vi "Action.vi"(8 "error in (no error)":errorcluster, 10 "Actor in":refnum<class "Tamagotchi Basic Actor.lvclass">, 11 "Sleep Message in":refnum<class "Sleep Message.lvclass">) -> (0 "error out":errorcluster, 2 "Actor out":refnum<class "Tamagotchi Basic Actor.lvclass">, 3 "Sleep Message out":refnum<class "Sleep Message.lvclass">)   [LabVIEW 2026, in "Sleep Message.lvclass"]
uses:
  Sleep Message.lvclass
  Tamagotchi Basic Actor/Tamagotchi Basic Actor.lvclass
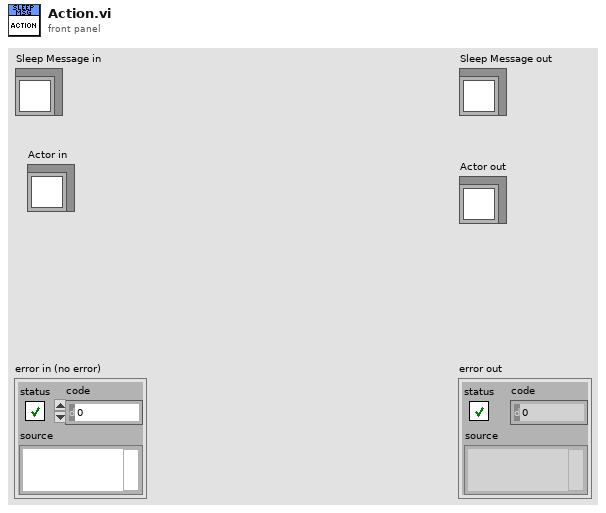
[diagram p1: front panel]
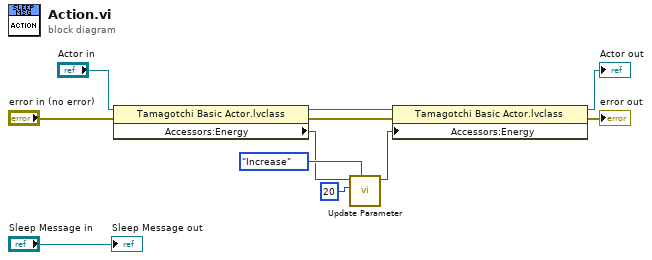
[diagram p0: block diagram]
diagram:
  n1 = property class="Tamagotchi Basic Actor.lvclass"(reference="Actor in", error in="error in (no error)") -> (reference out=w7:refnum<class "Tamagotchi Basic Actor.lvclass">, error out=w1:errorcluster, "Accessors:Energy"=w5:i16)
  n2 = call "Update Parameter.vi"("Action"=enum16{"Increase", "Decrease"}."Increase", "Modifier"=i16 20 ("y"), "Parameter"=w5) -> ("New Value"=w4:i16)  [unwired: 8 in]
  n3 = property class="Tamagotchi Basic Actor.lvclass"(reference=w7, error in=w1, "Accessors:Energy"=w4) -> (reference out=→"Actor out":refnum<class "Tamagotchi Basic Actor.lvclass">, error out=→"error out":errorcluster)
  "Sleep Message out" <- "Sleep Message in"
